vi "monitoring_sys_demo.vi"() -> ()   [LabVIEW 2023]
panel:
  in  "?":T1(tab)
  in  "?":bool
  out "?":bool
  out "Door's status":bool
  out "Oxygen Level [%]":dbl
  out "Temperture [C]":dbl
  out "Humidity [%]":dbl
  out "Waiting for Message":bool
  out "?":string
  out "Pressure Gauge 130B":picture caption="Liquid Nitrogen Tank Gauge"
  in  "?":bool
  out "Glove Box Panel_001 130B":picture caption="Glove Box Panel"
  out "string array":string[](array[string]) caption="Entry and Exit Data"
  in  "?":bool
  out "Message from Server":string
  out "Error Out":errorcluster caption="Error"
  out "Data from ESP32":dbl[](array[numeric])
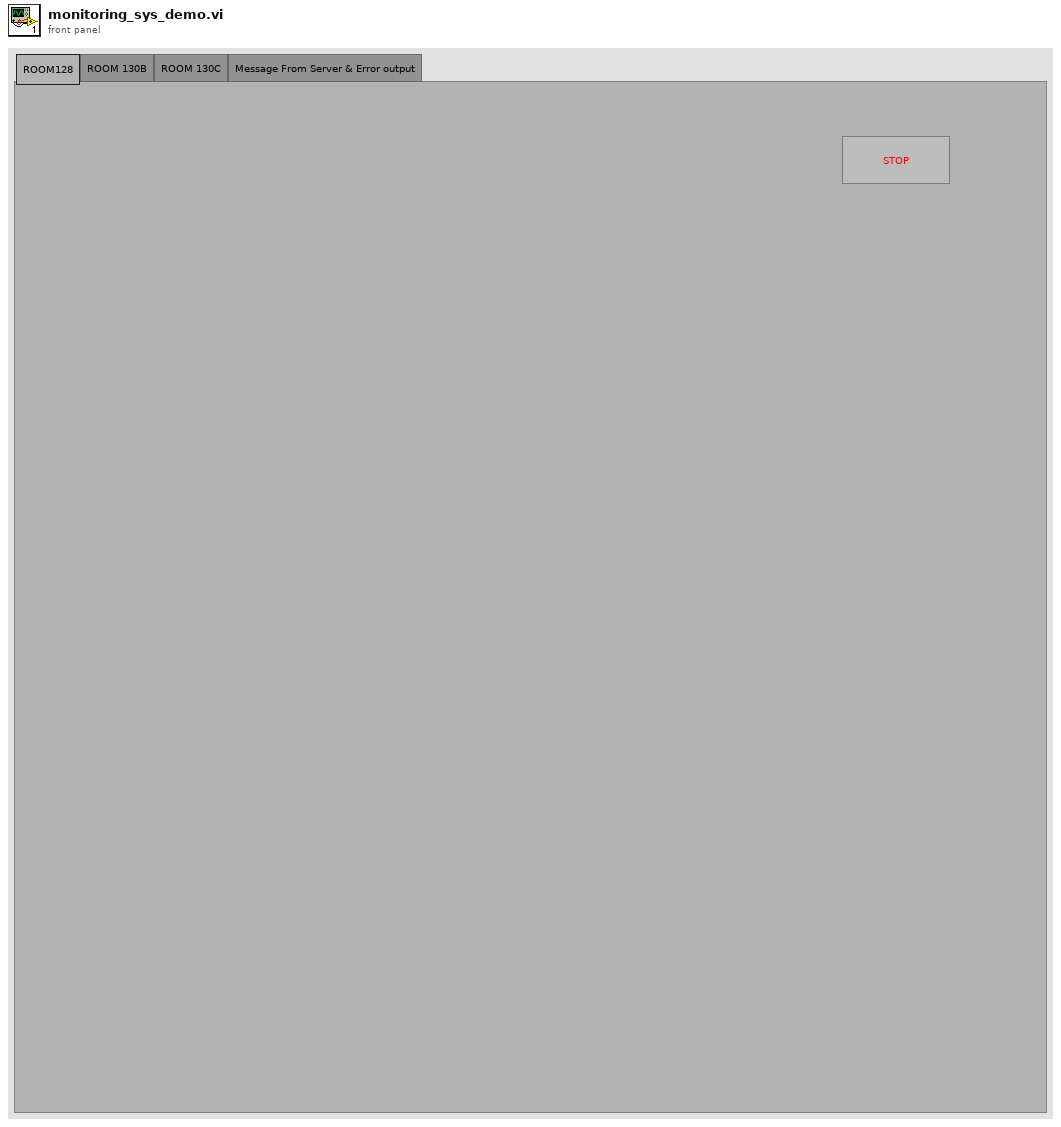
[diagram p1: front panel]
types:
  T1 = enum32{"ROOM128", "ROOM 130B", "ROOM 130C", "Message From Server & Error output"}
  T2 = enum16{"Standard", "Buffered", "CRLF", "Immediate"}
  T3 = typedef "imagedata.ctl" = cluster{"image type":i32, "image depth":i32, "image":u8[], "mask":u8[], "colors":u32[], "Rectangle":cluster{"left":i16, "top":i16, "right":i16, "bottom":i16}}
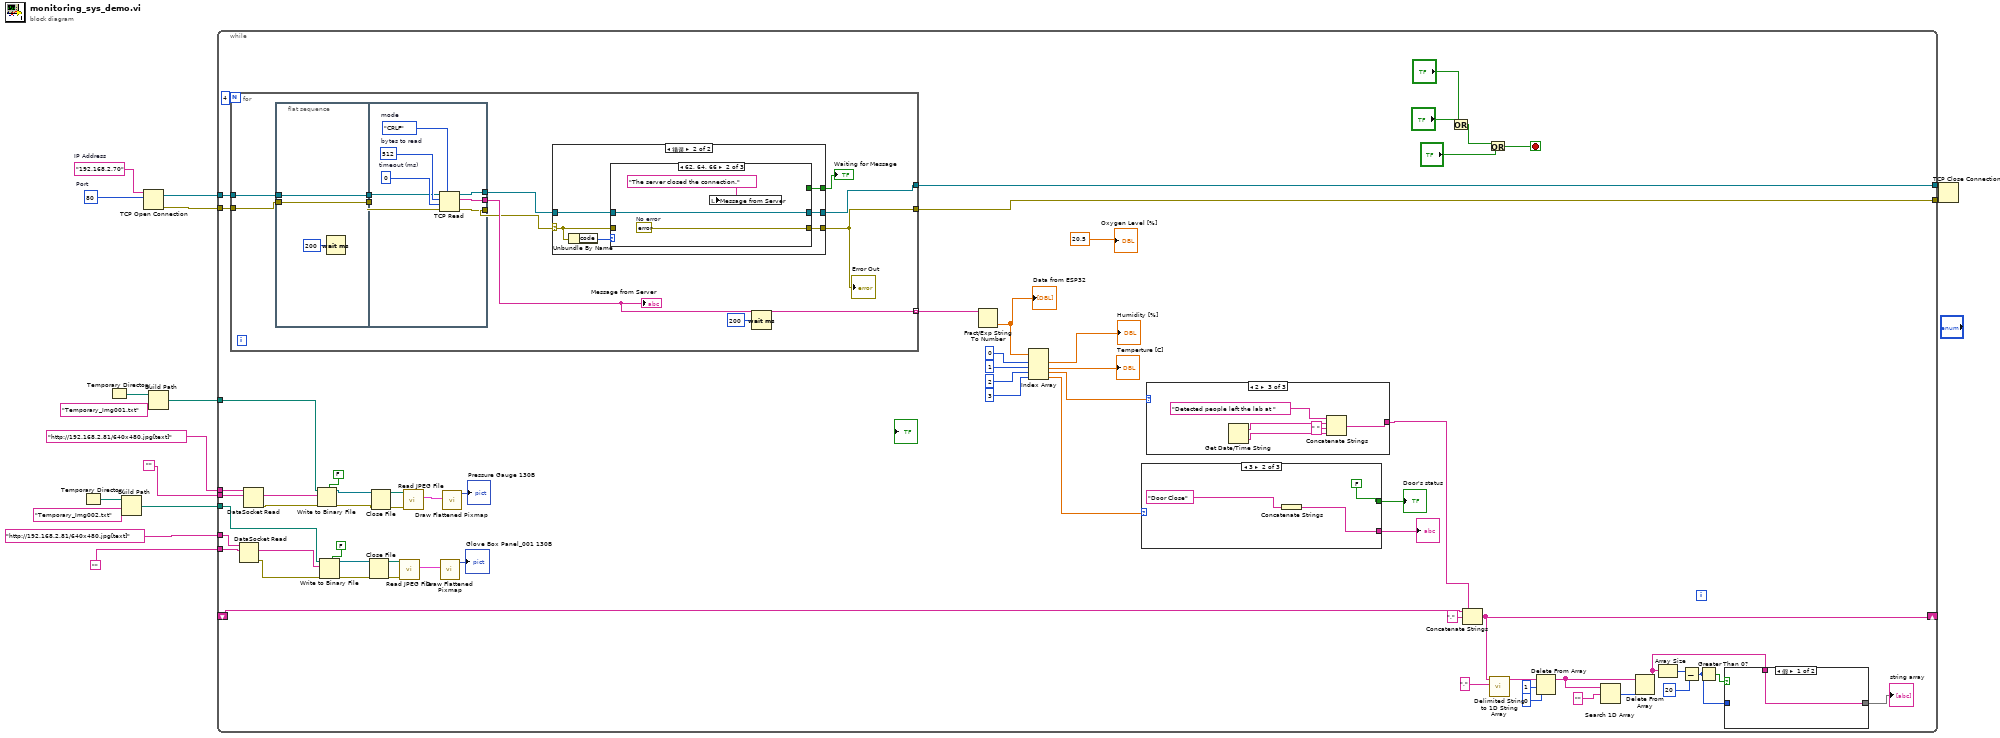
[diagram p0: block diagram]
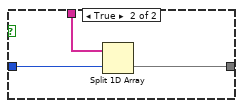
[diagram p2: hidden frame]
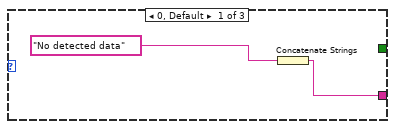
[diagram p3: hidden frame]
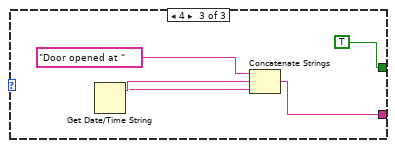
[diagram p4: hidden frame]
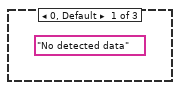
[diagram p5: hidden frame]
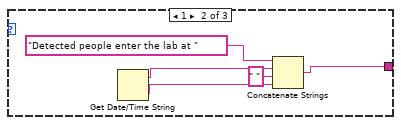
[diagram p6: hidden frame]
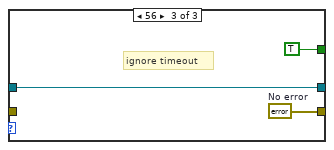
[diagram p9: hidden frame]
diagram:
  w15 = u16 80  # Port
  w16 = "192.168.2.70"  # IP Address
  n1 = Temporary Directory() -> (w3:path)
  n2 = Temporary Directory() -> (w6:path)
  n3 = Build Path(base path=w3, name or relative path="Temporary_Img002.txt") -> (appended path=w1:path)
  n4 = TCP Open Connection(address=w16, remote port or service name=w15) -> (connection ID=w14:refnum<k5>, error out=w13:errorcluster)  [unwired: 3 in]
  n5 = Build Path(base path=w6, name or relative path="Temporary_Img001.txt") -> (appended path=w4:path)
  n6 = while {
    tunnel: w14 -> [w79]
    tunnel: w13 -> [w78]
    tunnel: [w77] -> w12
    tunnel: [w76] -> w11
    tunnel: "http://192.168.2.81/640x480.jpg[text]" ("URL to JPG Image") -> [w42]
    tunnel: "" -> [w41]
    tunnel: "http://192.168.2.81/640x480.jpg[text]" ("URL to JPG Image") -> [w40]
    tunnel: "" -> [w39]
    shift-right: [w32] -> _
    shift-left: _ -> [w34]
    tunnel: w4 -> [w36]
    tunnel: w1 -> [w35]
    stop <- w52 stop-if-true
    n7 = for {
      N: 4 -> [_]
      tunnel: w79 -> [w113]
      tunnel: w78 -> [w112]
      tunnel: [w106] -> w77
      tunnel: [w105] -> w76
      tunnel: [w110] -> w75 mode=indexing
      n8 = flat-sequence {
        tunnel: w113 -> [w134]
        tunnel: [w134] -> w115
        tunnel: [w133] -> w114
        tunnel: w112 -> [w133]
        tunnel: [w139] -> w109
        tunnel: [w138] -> w110
        tunnel: [w137] -> w108
        tunnel: w115 -> [w136]
        tunnel: w114 -> [w135]
        frame #0 {
          n9 = Wait (ms)(milliseconds to wait=u32 200 ("等待时间（毫秒）")) -> ()  [unwired: 1 out]
        }
        frame #1 {
          w141 = 0  # timeout (ms)
          w142 = T2."CRLF"  # mode
          w140 = 512  # bytes to read
          n10 = TCP Read(connection ID=w136, bytes to read=w140, error in (no error)=w135, 7:w142, 9:w141) -> (connection ID out=w137:refnum<k5>, data out=w138:string, error out=w139:errorcluster)
        }
      }
      n11 = case shown="错误" w109 {
        selector: w109 -> [w117 w122]
        tunnel: [w117 w121] -> w105
        tunnel: w108 -> [w116 w120]
        tunnel: [w116 w119] -> w106
        tunnel: [_ w118] -> w107
        frame No Error {
        }
        frame Error {
          n12 = Unbundle By Name(w122) -> ("code"=w123:i32)
          n13 = case shown="62, 64, 66" w123 {
            tunnel: w122 -> [w125 _ _]
            tunnel: [w125 w128 w131] -> w121
            tunnel: [w124 w127 w130] -> w119
            tunnel: w120 -> [w124 w127 w130]
            tunnel: [_ _ TRUE] -> w118
            frame Default {
            }
            frame 62, 64, 66 {
              w128 = errorcluster {"status"=FALSE, "code"=0, "source"=""}  # No error
              n14 = local write "Message from Server"("The server closed the connection." ("Server Closed")) -> ()
            }
            frame 56 {
              w131 = errorcluster {"status"=FALSE, "code"=0, "source"=""}  # No error
              # "ignore timeout"
            }
          }
        }
      }
      "Waiting for Message" <- w107
      "Error Out" <- w105
      n15 = Wait (ms)(milliseconds to wait=u32 200) -> ()  [unwired: 1 out]
      "Message from Server" <- w110
    }
    n16 = DataSocket Read(10:w41, 11:w42) -> (0:w43:errorcluster, 2:w44:string)  [unwired: 1 in, 7 out]
    n17 = DataSocket Read(10:w39, 11:w40) -> (0:w37:errorcluster, 2:w38:string)  [unwired: 1 in, 7 out]
    n18 = Write to Binary File(file (use dialog)=w36, data=w38, error in=w37, 5:FALSE ("prepend array or string size? (T)")) -> (refnum out=w48:refnum<file>, error out=w47:errorcluster)  [unwired: 3 out]
    n19 = Write to Binary File(file (use dialog)=w35, data=w44, error in=w43, 5:FALSE ("prepend array or string size? (T)")) -> (refnum out=w46:refnum<file>, error out=w45:errorcluster)  [unwired: 3 out]
    n20 = Close File(refnum=w46, error in=w45) -> (path=w58:path, error out=w60:errorcluster)
    n21 = Close File(refnum=w48, error in=w47) -> (path=w62:path, error out=w63:errorcluster)
    n22 = call <vilib>:"Read JPEG File.vi"("error in (no error)"=w60, "path to JPEG file"=w58) -> ("image data"=w59:T3)  [unwired: 7 in, 2 out]
    n23 = call <vilib>:"Read JPEG File.vi"("error in (no error)"=w63, "path to JPEG file"=w62) -> ("image data"=w51:T3)  [unwired: 9 out]
    n24 = call <vilib>:"Draw Flattened Pixmap.vi"("image data"=w59) -> ("new picture"=→"Glove Box Panel_001 130B":picture)  [unwired: 1 in, 7 out]
    n25 = call <vilib>:"Draw Flattened Pixmap.vi"("image data"=w51) -> ("new picture"=→"Pressure Gauge 130B":picture)  [unwired: 1 in, 7 out]
    n26 = Fract/Exp String To Number(string=w75) -> (number=w72:dbl[])  [unwired: 3 in, 1 out]
    "Data from ESP32" <- w72
    n27 = Index Array(array=w72, index #1=0 ("索引"), index #2=1 ("索引"), index #3=2 ("索引"), index #4=3 ("索引")) -> (element #1=→"Humidity [%]":dbl, element #2=→"Temperture [C]":dbl, element #3=w67:dbl, element #4=w66:dbl)
    n28 = case shown="3" w66 {
      tunnel: [_ FALSE TRUE] -> w65
      tunnel: [w85 w87 w90] -> w33
      frame 0, Default {
        n29 = Concatenate Strings("No detected data") -> (w85:string)
      }
      frame 3 {
        n30 = Concatenate Strings("Door Close") -> (w87:string)
      }
      frame 4 {
        n31 = Get Date/Time String() -> (date string=w94:string, time string=w93:string)  [unwired: 3 in]
        n32 = Concatenate Strings("Door opened at ", w94, w93) -> (w90:string)
      }
    }
    "Door's status" <- w65
    "?" <- w33
    n33 = case shown="2" w67 {
      tunnel: [_ w97 w102] -> w30
      frame 0, Default {
        (unwired) "No detected data"
      }
      frame 1 {
        n34 = Get Date/Time String() -> (date string=w98:string, time string=w96:string)  [unwired: 3 in]
        n35 = Concatenate Strings("Detected people enter the lab at ", w98, " " ("字符串"), w96) -> (w97:string)
      }
      frame 2 {
        n36 = Get Date/Time String() -> (date string=w104:string, time string=w101:string)  [unwired: 3 in]
        n37 = Concatenate Strings("Detected people left the lab at ", w104, " " ("字符串"), w101) -> (w102:string)
      }
    }
    n38 = Or(x="?", y="?") -> (x .or. y?=w54:bool)
    n39 = Concatenate Strings(w34, "," ("字符串"), w30) -> (w32:string)
    n40 = Or(x=w54, y="?") -> (x .or. y?=w52:bool)
    n41 = call <vilib>:"Delimited String to 1D String Array.vi"("delimiter"=",", "delimited string"=w32) -> ("string array"=w28:string[])  [unwired: 9 in]
    n42 = Delete From Array(array=w28, length=1 ("长度"), index=0 ("索引")) -> (array with subset deleted=w24:string[])  [unwired: 1 out]
    n43 = Search 1D Array(1D array=w24, element="" ("元素")) -> (index of element=w23:i32)  [unwired: 1 in]
    n44 = Delete From Array(array=w24, index=w23) -> (array with subset deleted=w19:string[])  [unwired: 1 in, 1 out]
    n45 = Array Size(array=w19) -> (size(s)=w22:i32)
    n46 = Subtract(x=w22, y=20) -> (x-y=w18:i32)
    n47 = Greater Than 0?(x=w18) -> (x > 0?=w20:bool)
    n48 = case shown="假" w20 {
      tunnel: w19 -> [w81 w84]
      tunnel: w18 -> [_ w83]
      tunnel: [w81 w82] -> w17
      frame False {
      }
      frame True {
        n49 = Split 1D Array(array=w84, index=w83) -> (second subarray=w82:string[])  [unwired: 1 out]
      }
    }
    "string array" <- w17
    "Oxygen Level [%]" <- 20.5 ("Oxygen Level")
  }
  n50 = TCP Close Connection(connection ID=w12, error in (no error)=w11) -> ()  [unwired: 3 out]
